vi "2700电流加载及换向回读-PLC.vi"(0 "6510 in":refnum<visa-resource-name>, 1 "TDK in":refnum<visa-resource-name>, 2 "输入电流":dbl, 3 "Delay Time (s)":dbl=1.0 caption="延迟时间(s)", 4 "电源台数":u8=1, 5 "error in":errorcluster, 7 "y":dbl=5000.0 format="%#_13g") -> (6 "IsSuccess":bool, 14 "2700 out":refnum<visa-resource-name>, 15 "TDK out":refnum<visa-resource-name>, 16 "实际电流":dbl, 19 "error out":errorcluster)   [LabVIEW 2020]
uses:
  HslCommunication.dll
  <instrlib>/Keithley 27XX/Public/Data/Read Single Point.vi
  <instrlib>/TDK-Lambda G Series/TDK-Lambda G Series.lvlib
  <instrlib>/Keithley 27XX/Keithley 27XX.lvlib
panel:
  out "x*y":dbl
  # "TDK 电流加载及换向"
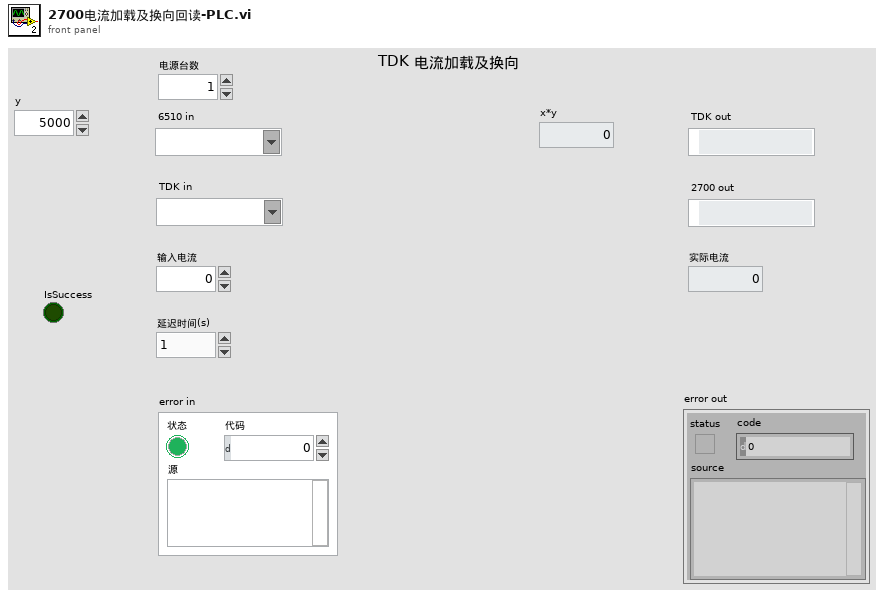
[diagram p1: front panel]
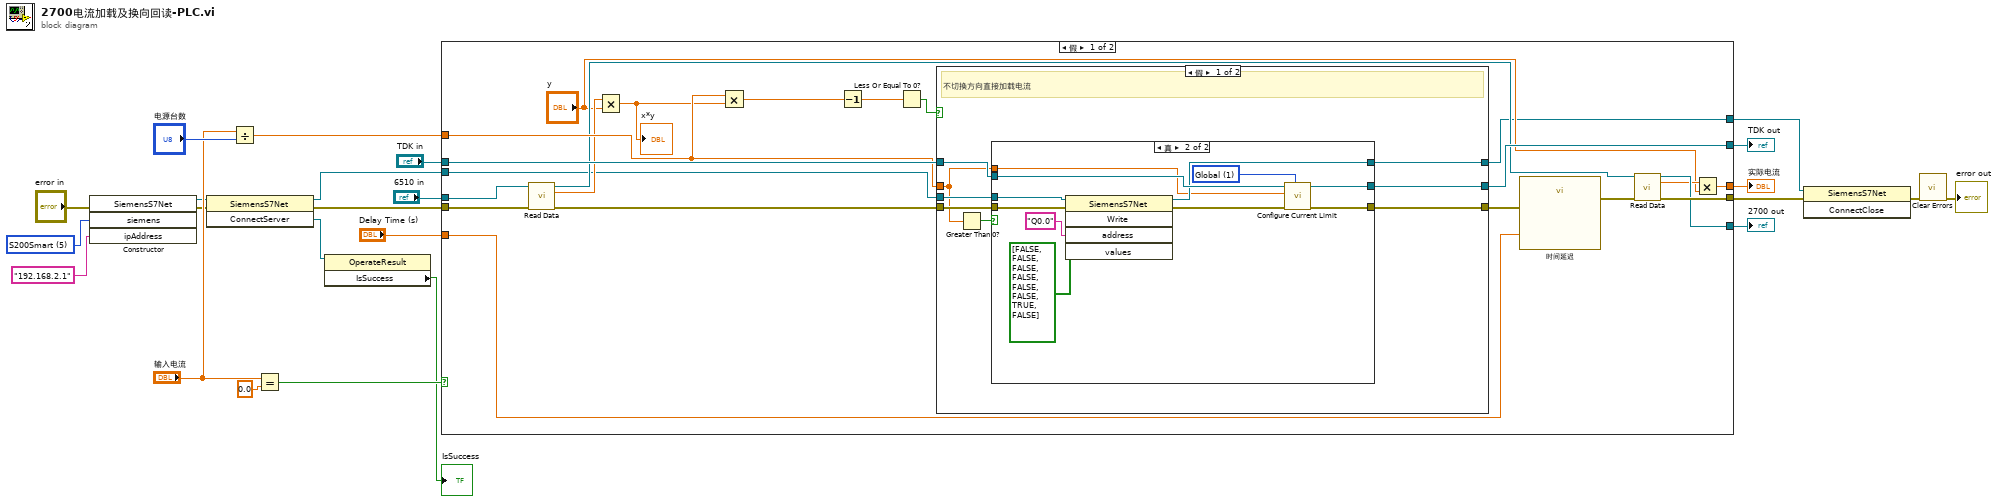
[diagram p0: block diagram]
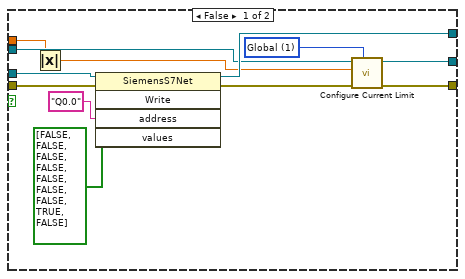
[diagram p2: hidden frame]
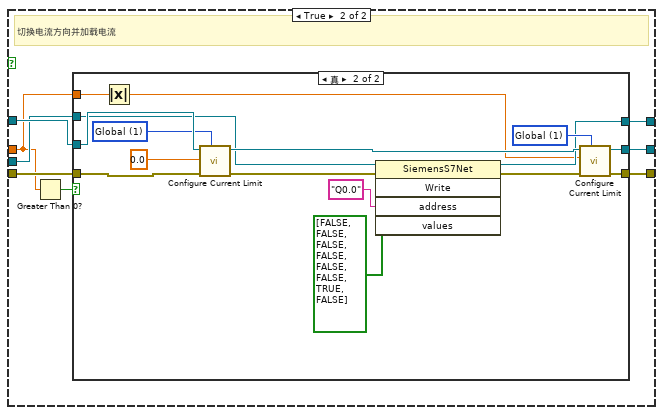
[diagram p3: hidden frame]
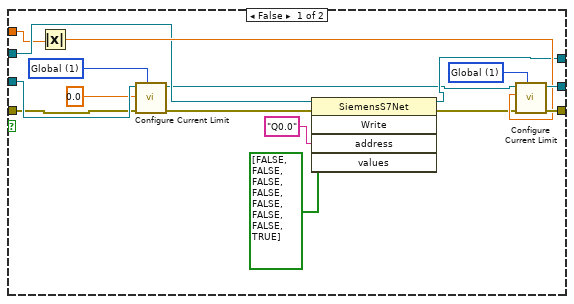
[diagram p4: hidden frame]
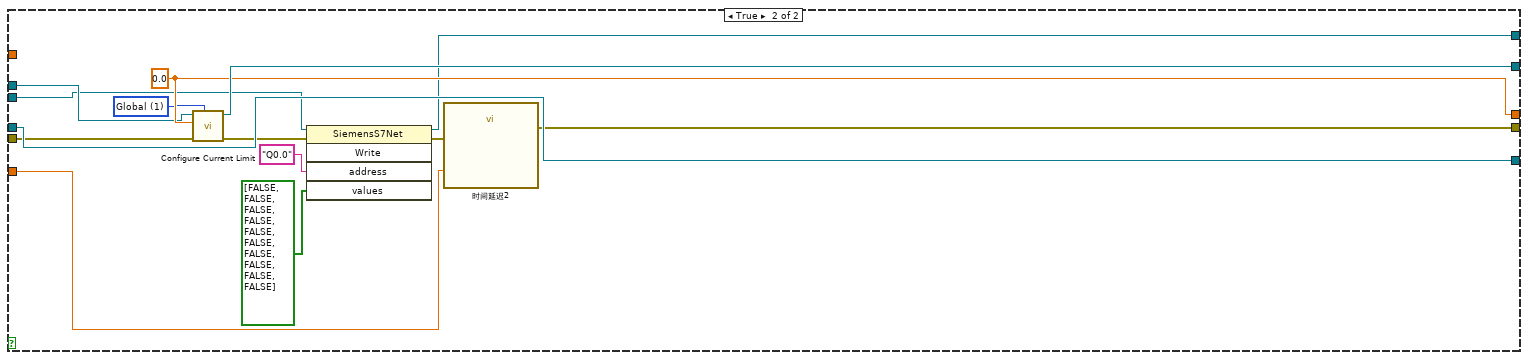
[diagram p5: hidden frame]
diagram:
  w12 = 5 items=["S1200"=1, "S300"=2, "S400"=3, "S1500"=4, "S200Smart"=5, "S200"=6] ("siemens")
  n1 = constructor class="SiemensS7Net"(error in="error in", "siemens"=w12, "ipAddress"="192.168.2.1") -> (reference out=w9:refnum<k24>, error out=w10:errorcluster)  [unwired: 2 in, 3 out]
  n2 = invoke class="SiemensS7Net" method="ConnectServer"(reference=w9, error in=w10) -> (reference out=w6:refnum<k24>, error out=w3:errorcluster, "ConnectServer"=w8:refnum<k24>)  [unwired: 1 in]
  n3 = Divide(x="输入电流", y="电源台数") -> (x/y=w14:dbl)
  n4 = Equal?(x="输入电流", y=0.0) -> (x = y?=w20:bool)
  n5 = property class="OperateResult"(reference=w8) -> ("IsSuccess"=→"IsSuccess":bool)  [unwired: 1 in, 2 out]
  n6 = case shown="假" w20 {
    tunnel: "TDK in" -> [w43 w127]
    tunnel: [w30 w125] -> w2
    tunnel: "Delay Time (s)" -> [w41 w124]
    tunnel: w3 -> [w34 w129]
    tunnel: [w40 w130] -> w22
    tunnel: "6510 in" -> [w35 w131]
    tunnel: [w29 w131] -> w18
    tunnel: w14 -> [w39 _]
    tunnel: [w37 w128] -> w19
    tunnel: w6 -> [w26 w121]
    tunnel: [w25 w120] -> w5
    frame False {
      n7 = call-poly <instrlib>:"Read Data.vi"("VISA resource name"=w35, "error in (no error)"=w34) -> ("VISA resource name out"=w32:refnum<visa-resource-name>, "Measurement Data"=w36:dbl, "error out"=w33:errorcluster)  [unwired: 11 in]
      n8 = Multiply(x=w36, y="y") -> (x*y=w38:dbl)
      "x*y" <- w38
      n9 = Multiply(x=w39, y=w38) -> (x*y=w45:dbl)
      n10 = Decrement(x=w45) -> (x-1=w44:dbl)
      n11 = Less Or Equal To 0?(x=w44) -> (x <= 0?=w46:bool)
      n12 = case shown="假" w46 {
        tunnel: w39 -> [w47 w78]
        tunnel: w33 -> [w51 w82]
        tunnel: w43 -> [w53 w84]
        tunnel: [w52 w83] -> w42
        tunnel: [w50 w81] -> w40
        tunnel: w26 -> [w48 w80]
        tunnel: [w49 w79] -> w25
        frame False {
          # "不切换方向直接加载电流"
          n13 = Greater Than 0?(x=w47) -> (x > 0?=w54:bool)
          n14 = case shown="真" w54 {
            tunnel: w53 -> [w59 w76]
            tunnel: [w65 w75] -> w52
            tunnel: w51 -> [w58 w73]
            tunnel: [w66 w77] -> w50
            tunnel: [w62 w71] -> w49
            tunnel: w48 -> [w60 w68]
            tunnel: w47 -> [w56 w67]
            frame False {
              w64 = u16 1 items=["Single", "Global"] ("Globalize (0: Single)")
              n15 = Absolute Value(x=w56) -> (abs(x)=w55:dbl)
              n16 = invoke class="SiemensS7Net" method="Write"(reference=w60, error in=w58, "address"="Q0.0", "values"=bool[] [FALSE, FALSE, FALSE, FALSE, FALSE, FALSE, FALSE, TRUE, FALSE]) -> (reference out=w62:refnum<k24>, error out=w63:errorcluster)  [unwired: 1 in, 3 out]
              n17 = call <instrlib>:"Configure Current Limit.vi"("Globalize (0: Single)"=w64, "error in (no error)"=w63, "Current Limit (0A)"=w55, "VISA resource name"=w59) -> ("error out"=w65:errorcluster, "VISA resource name out"=w66:refnum<visa-resource-name>)  [unwired: 6 in]
            }
            frame True {
              w74 = u16 1 items=["Single", "Global"] ("Globalize (0: Single)")
              n18 = invoke class="SiemensS7Net" method="Write"(reference=w68, error in=w73, "address"="Q0.0", "values"=bool[] [FALSE, FALSE, FALSE, FALSE, FALSE, FALSE, TRUE, FALSE]) -> (reference out=w71:refnum<k24>, error out=w72:errorcluster)  [unwired: 1 in, 3 out]
              n19 = call <instrlib>:"Configure Current Limit.vi"("Globalize (0: Single)"=w74, "error in (no error)"=w72, "Current Limit (0A)"=w67, "VISA resource name"=w76) -> ("error out"=w75:errorcluster, "VISA resource name out"=w77:refnum<visa-resource-name>)  [unwired: 6 in]
            }
          }
        }
        frame True {
          # "切换电流方向并加载电流"
          n20 = Greater Than 0?(x=w78) -> (x > 0?=w85:bool)
          n21 = case shown="真" w85 {
            tunnel: w84 -> [w98 w115]
            tunnel: [w101 w117] -> w83
            tunnel: w82 -> [w96 w113]
            tunnel: [w100 w116] -> w81
            tunnel: w80 -> [w93 w105]
            tunnel: [w92 w106] -> w79
            tunnel: w78 -> [w86 w103]
            frame False {
              w94 = u16 1 items=["Single", "Global"] ("Globalize (0: Single)")
              w95 = u16 1 items=["Single", "Global"] ("Globalize (0: Single)")
              n22 = Absolute Value(x=w86) -> (abs(x)=w99:dbl)
              n23 = call <instrlib>:"Configure Current Limit.vi"("Globalize (0: Single)"=w94, "error in (no error)"=w96, "Current Limit (0A)"=0.0 ("Curr(0)"), "VISA resource name"=w98) -> ("error out"=w91:errorcluster, "VISA resource name out"=w88:refnum<visa-resource-name>)  [unwired: 6 in]
              n24 = invoke class="SiemensS7Net" method="Write"(reference=w93, error in=w91, "address"="Q0.0", "values"=bool[] [FALSE, FALSE, FALSE, FALSE, FALSE, FALSE, FALSE, TRUE]) -> (reference out=w92:refnum<k24>, error out=w90:errorcluster)  [unwired: 1 in, 3 out]
              n25 = call <instrlib>:"Configure Current Limit.vi"("Globalize (0: Single)"=w95, "error in (no error)"=w90, "Current Limit (0A)"=w99, "VISA resource name"=w88) -> ("error out"=w101:errorcluster, "VISA resource name out"=w100:refnum<visa-resource-name>)  [unwired: 6 in]
            }
            frame True {
              w110 = u16 1 items=["Single", "Global"] ("Globalize (0: Single)")
              w111 = u16 1 items=["Single", "Global"] ("Globalize (0: Single)")
              n26 = Absolute Value(x=w103) -> (abs(x)=w102:dbl)
              n27 = call <instrlib>:"Configure Current Limit.vi"("Globalize (0: Single)"=w110, "error in (no error)"=w113, "Current Limit (0A)"=0.0 ("Curr(0)"), "VISA resource name"=w115) -> ("error out"=w109:errorcluster, "VISA resource name out"=w112:refnum<visa-resource-name>)  [unwired: 6 in]
              n28 = invoke class="SiemensS7Net" method="Write"(reference=w105, error in=w109, "address"="Q0.0", "values"=bool[] [FALSE, FALSE, FALSE, FALSE, FALSE, FALSE, TRUE, FALSE]) -> (reference out=w106:refnum<k24>, error out=w108:errorcluster)  [unwired: 1 in, 3 out]
              n29 = call <instrlib>:"Configure Current Limit.vi"("Globalize (0: Single)"=w111, "error in (no error)"=w108, "Current Limit (0A)"=w102, "VISA resource name"=w112) -> ("error out"=w117:errorcluster, "VISA resource name out"=w116:refnum<visa-resource-name>)  [unwired: 6 in]
            }
          }
        }
      }
      n30 = call "时间延迟"("error in (no error)"=w42, "Delay Time (s)"=w41) -> ("error out"=w31:errorcluster)  [unwired: 9 in]
      n31 = call-poly <instrlib>:"Read Data.vi"("VISA resource name"=w32, "error in (no error)"=w31) -> ("VISA resource name out"=w29:refnum<visa-resource-name>, "Measurement Data"=w28:dbl, "error out"=w30:errorcluster)  [unwired: 11 in]
      n32 = Multiply(x=w28, y="y") -> (x*y=w37:dbl)
    }
    frame True {
      w126 = u16 1 items=["Single", "Global"] ("Globalize (0: Single)")
      w128 = 0.0 ("Curr(0)")
      n33 = call <instrlib>:"Configure Current Limit.vi"("Globalize (0: Single)"=w126, "error in (no error)"=w129, "Current Limit (0A)"=w128, "VISA resource name"=w127) -> ("error out"=w122:errorcluster, "VISA resource name out"=w130:refnum<visa-resource-name>)  [unwired: 6 in]
      n34 = invoke class="SiemensS7Net" method="Write"(reference=w121, error in=w122, "address"="Q0.0", "values"=bool[] [FALSE, FALSE, FALSE, FALSE, FALSE, FALSE, FALSE, FALSE, FALSE, FALSE]) -> (reference out=w120:refnum<k24>, error out=w123:errorcluster)  [unwired: 1 in, 3 out]
      n35 = call "时间延迟2"("error in (no error)"=w123, "Delay Time (s)"=w124) -> ("error out"=w125:errorcluster)  [unwired: 9 in]
    }
  }
  "实际电流" <- w19
  "TDK out" <- w22
  "2700 out" <- w18
  n36 = invoke class="SiemensS7Net" method="ConnectClose"(reference=w5, error in=w2) -> (error out=w1:errorcluster)  [unwired: 1 in, 2 out]
  n37 = call <vilib>:"Clear Errors.vi"("error in (no error)"=w1) -> ("error out"=→"error out":errorcluster)  [unwired: 5 in, 1 out]
